vi "Register Message Metadata.vi"(8 "error in (no error)":errorcluster, 10 "Messages":T2[](array[typedef]), 11 "gRPCid":T1) -> (0 "error out":errorcluster, 3 "gRPCid":T1)   [LabVIEW 2019, in "gprc-lvsupport.lvlib"]
uses:
  gprc-lvsupport.lvlib
  typeDefs/Message Metadata.ctl
  typeDefs/Message Element Metadata.ctl
  typeDefs/Message Element Type.ctl
  typeDefs/grpcId.ctl
  dlls/labview_grpc_server.dll
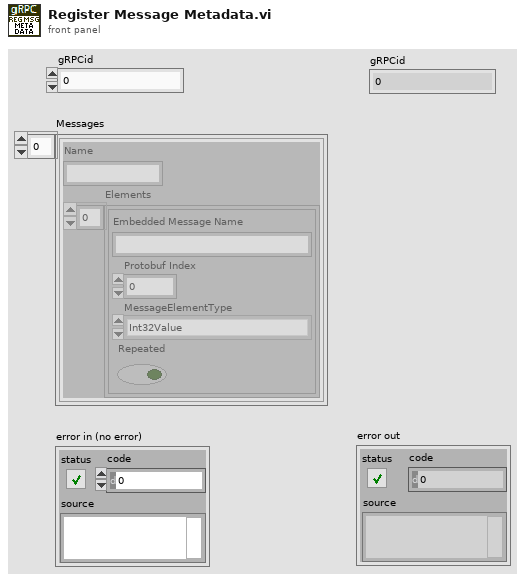
[diagram p1: front panel]
types:
  T1 = typedef "gprc-lvsupport.lvlib/grpcId.ctl" = u64
  T2 = typedef "gprc-lvsupport.lvlib/Message Metadata.ctl" = cluster{"Name":string, "Elements":T3[]}
  T3 = typedef "gprc-lvsupport.lvlib/Message Element Metadata.ctl" = cluster{"Embedded Message Name":string, "Protobuf Index":i32, "MessageElementType":T4, "Repeated":bool}
  T4 = typedef "gprc-lvsupport.lvlib/Message Element Type.ctl" = enum32{"Int32Value", "FloatValue", "DoubleValue", "BoolValue", "StringValue", "MessageValue", ""}
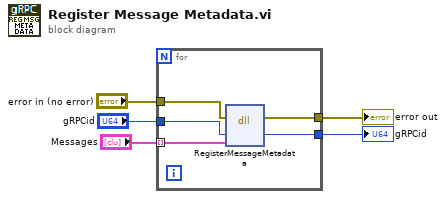
[diagram p0: block diagram]
diagram:
  n1 = for {
    tunnel: "Messages" -> [w10] mode=indexing
    tunnel: "gRPCid" -> [w9]
    tunnel: "error in (no error)" -> [w8]
    tunnel: [w7] -> w2
    tunnel: [w6] -> w1
    n2 = dll-call lib="C:/Users/XEnderMD/Desktop/LV gRPC/labview source/gRPC interface/dlls/labview_grpc_server.dll" fn="RegisterMessageMetadata"(error in=w8, w9, "metadata"=w10) -> (error out=w7:errorcluster, w6:T1)  [unwired: 4 in, 1 out]
  }
  "error out" <- w2
  "gRPCid" <- w1
